vi "Autonomous Independent.vi"   [LabVIEW 2011]
doc: "This VI is called when autonomous begins, and will automatically be terminated when autonomous ends. You can carry out timed or sensor driven robot movement independently without needing to return to the caller."
uses:
  <vilib>/Rock Robotics/WPI/SafetyOutput/WPI_SafetyOutputConfigMenu.ctl
  Robot Global Data.vi
  System Set Points and States.vi
types:
  T1 = typedef "WPI_SafetyOutputConfigMenu.ctl" = enum16{"Enable", "Disable"}
  T2 = typedef "WPI_MotorControlDeviceRef.ctl" = cluster{"DeviceStatus":errorcluster, "Type":enum16{"PWM", "CAN"}, "PWM":cluster{"Digital Module":T3, "PWM Channel":T4, "DeadBand":T5}, "CAN":cluster{"Device Number":u8, "Control Mode":T6, "Semaphore":T7, "Max Vout":dbl}, "Invert":bool, "TransformRef":T8, "InvTransformRef":T8}
  T3 = typedef "FPGA_TypedefDigitalModule.ctl" = enum16{"Digital Module 1", "Digital Module 2"}
  T4 = typedef "FPGA_DIOPWMChannel.ctl" = enum8{"PWM 1", "PWM 2", "PWM 3", "PWM 4", "PWM 5", "PWM 6", "PWM 7", "PWM 8", "PWM 9", "PWM 10", "Invalid"}
  T5 = typedef "WPI_PWMDeadband.ctl" = cluster{"Name":string, "maxPositivePwm":i32, "minPositivePwm":i32, "centerPwm":i32, "maxNegativePwm":i32, "minNegativePwm":i32, "angularRange":u16}
  T6 = typedef "WPI_CANJaguar_ControlMode.ctl" = enum8{"Percent VBus", "Current", "Speed", "Position", "Voltage"}
  T7 = typedef "Semaphore RefNum" = refnum<k1>
  T8 = typedef "WPI_PWMTransform_ConPane.ctl" = refnum<vi>
  T9 = typedef "WPI_DigitalInputDevRef.ctl" = cluster{"DevStatus":errorcluster, "DIO Channel":T10, "Digital Module":T3}
  T10 = typedef "FPGA_DIOChannel.ctl" = enum8{"DIO 1", "DIO 2", "DIO 3", "DIO 4", "DIO 5", "DIO 6", "DIO 7", "DIO 8", "DIO 9", "DIO 10", "DIO 11", "DIO 12", "DIO 13", "DIO 14", "Invalid"}
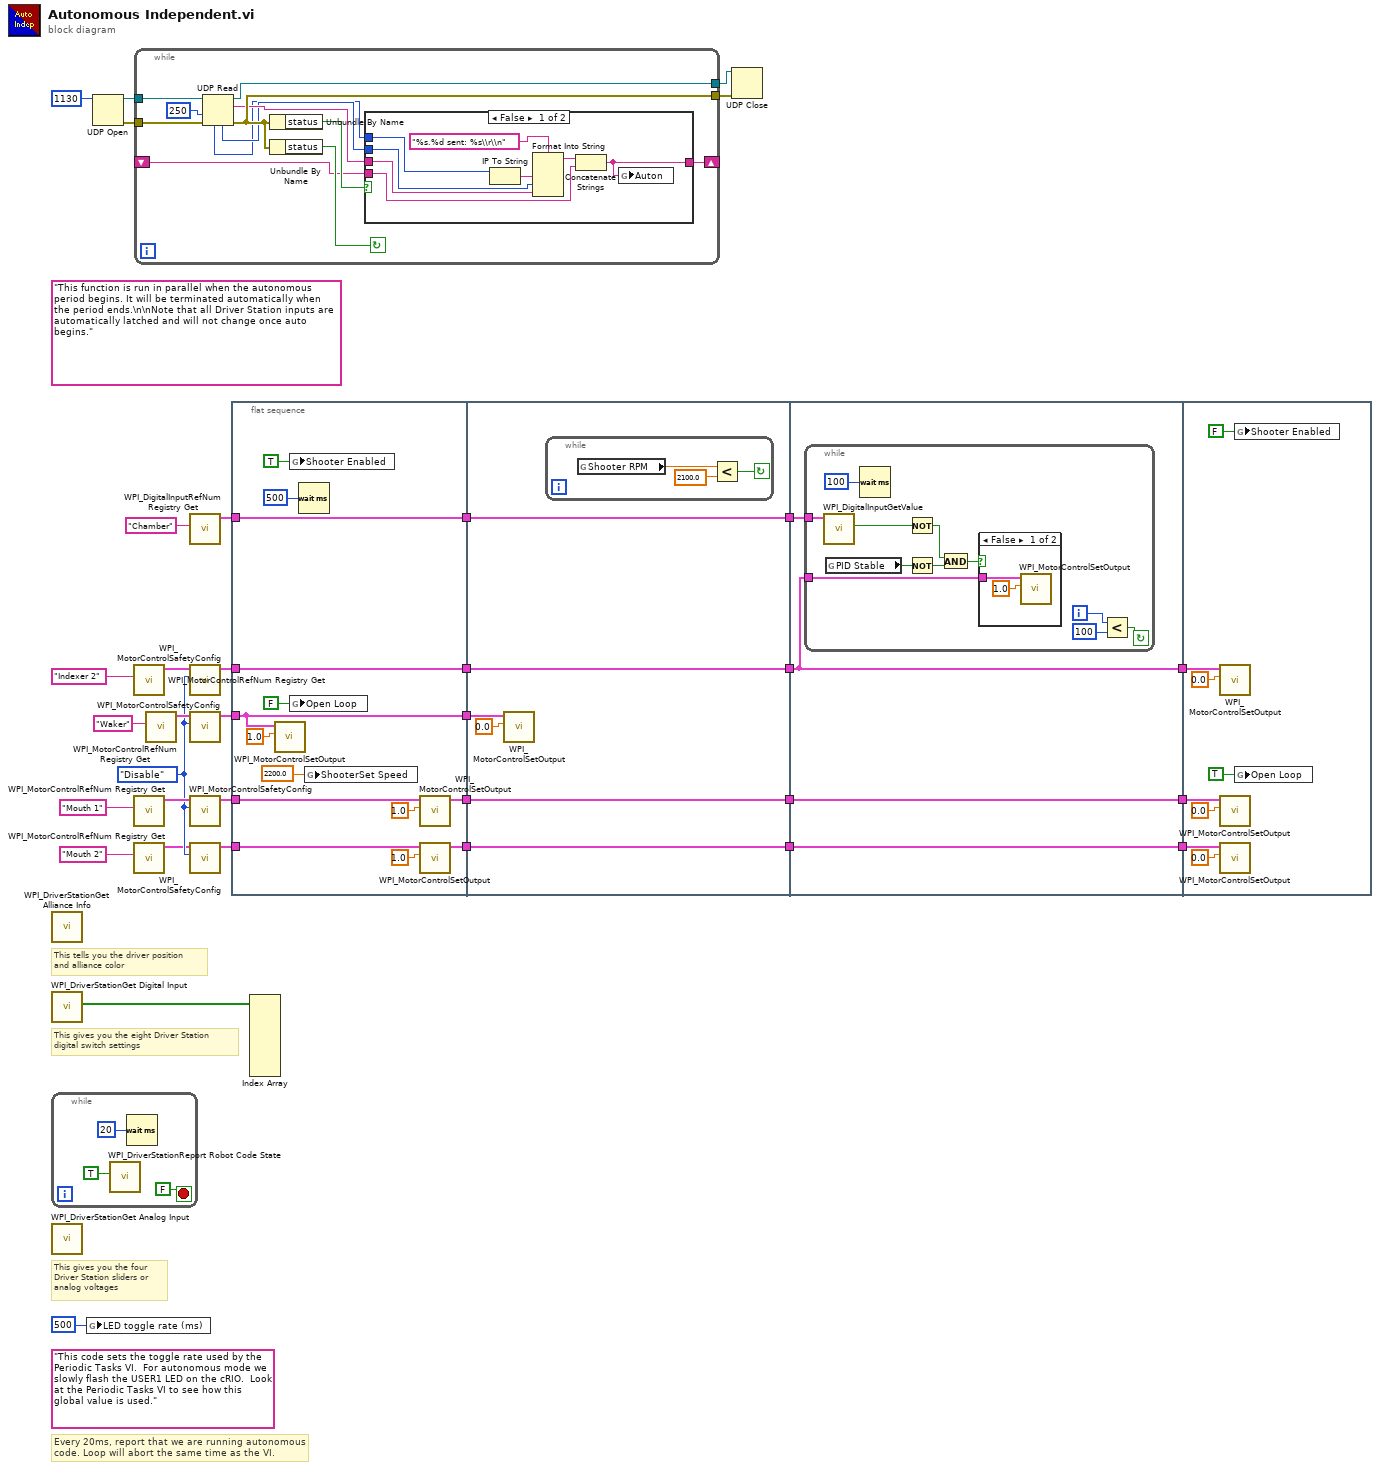
[diagram p0: block diagram]
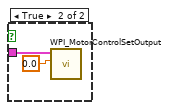
[diagram p2: hidden frame]
diagram:
  w6 = WPI_SafetyOutputConfigMenu."Disable" ("mode")
  (unwired) "This code sets the toggle rate used by the Periodic Tasks VI.  For autonomous mode we slowly flash the USER1 LED on the cRIO.  Look at the Periodic Tasks VI to see how this global value is used."
  (unwired) "This function is run in parallel when the autonomous period begins. It will be terminated automatically when the period ends.\n\nNote that all Driver Station inputs are automatically latched and will not change once auto begins."
  # "Every 20ms, report that we are running autonomous\ncode. Loop will abort the same time as the VI."
  # "This tells you the driver position\nand alliance color"
  # "This gives you the eight Driver Station\ndigital switch settings"
  # "This gives you the four\nDriver Station sliders or\nanalog voltages"
  n1 = call <vilib>:"WPI_DriverStationGet Alliance Info.vi"() -> ()  [unwired: 12 out]
  n2 = call <vilib>:"WPI_DriverStationGet Digital Input.vi"() -> ("Driver Station Digital Input (1-8)"=w20:bool[])  [unwired: 11 out]
  n3 = while {
    stop <- FALSE stop-if-true
    n4 = call <vilib>:"WPI_DriverStationReport Robot Code State.vi"("Autonomous"=TRUE) -> ()  [unwired: 10 in, 1 out]
    n5 = Wait (ms)(milliseconds to wait=u32 20) -> ()  [unwired: 1 out]
  }
  n6 = call <vilib>:"WPI_DriverStationGet Analog Input.vi"() -> ()  [unwired: 12 out]
  n7 = global write "Robot Global Data.vi" "LED toggle rate (ms)"(u32 500 ("LED ms toggle rate")) -> ()
  n8 = UDP Open(11:u16 1130 ("port")) -> (port=w32:refnum<k16>, 0:w34:errorcluster)  [unwired: 4 in, 1 out]
  n9 = call <vilib>:"WPI_MotorControlRefNum Registry Get.vi"("refnum name"="Indexer 2") -> ("MotorControlDevRef"=w16:T2)  [unwired: 9 in, 1 out]
  n10 = call <vilib>:"WPI_MotorControlRefNum Registry Get.vi"("refnum name"="Mouth 1") -> ("MotorControlDevRef"=w11:T2)  [unwired: 9 in, 1 out]
  n11 = call <vilib>:"WPI_MotorControlRefNum Registry Get.vi"("refnum name"="Mouth 2") -> ("MotorControlDevRef"=w5:T2)  [unwired: 9 in, 1 out]
  n12 = while {
    tunnel: w34 -> [w49]
    tunnel: w32 -> [w48]
    tunnel: [w47] -> w31
    tunnel: [w44] -> w30
    shift-right: [w38] -> _
    shift-left: _ -> [w39]
    stop <- w45 continue-if-true
    n13 = UDP Read(connection ID=w48, timeout ms (25000)=250, 8:w49) -> (data out=w42:string, error out=w44:errorcluster, 3:w47:refnum<k16>, 4:w41:u16, 6:w40:u32)  [unwired: 1 in]
    n14 = Unbundle By Name(w44) -> ("status"=w43:bool)
    n15 = Unbundle By Name(w44) -> ("status"=w45:bool)
    n16 = case shown="False" w43 {
      tunnel: w42 -> [w51 _]
      tunnel: w41 -> [w55 _]
      tunnel: w40 -> [w53 _]
      tunnel: w39 -> [w52 w58]
      tunnel: [w50 w58] -> w38
      frame False {
        n17 = IP To String(2:w53) -> (0:w54:string)  [unwired: 1 in]
        n18 = Format Into String(format string="%s.%d sent: %s\\r\\n", w54, w55, w51) -> (resulting string=w57:string)  [unwired: 2 in, 1 out]
        n19 = Concatenate Strings(w57, w52) -> (w50:string)
        n20 = global write "System Set Points and States.vi" "Auton"(w50) -> ()
      }
      frame True {
      }
    }
  }
  n21 = call <vilib>:"WPI_MotorControlRefNum Registry Get.vi"("refnum name"="Waker") -> ("MotorControlDevRef"=w14:T2)  [unwired: 9 in, 1 out]
  n22 = call <vilib>:"WPI_DigitalInputRefNum Registry Get.vi"("refnum name"="Chamber") -> ("DigitalInputDevRef"=w12:T9)  [unwired: 9 in, 1 out]
  n23 = call <vilib>:"WPI_MotorControlSafetyConfig.vi"("mode"=w6, "MotorControlDevRef"=w16) -> ("MotorControlDevRef"=w15:T2)  [unwired: 8 in, 1 out]
  n24 = call <vilib>:"WPI_MotorControlSafetyConfig.vi"("mode"=w6, "MotorControlDevRef"=w14) -> ("MotorControlDevRef"=w13:T2)  [unwired: 8 in, 1 out]
  n25 = call <vilib>:"WPI_MotorControlSafetyConfig.vi"("mode"=w6, "MotorControlDevRef"=w11) -> ("MotorControlDevRef"=w9:T2)  [unwired: 8 in, 1 out]
  n26 = call <vilib>:"WPI_MotorControlSafetyConfig.vi"("mode"=w6, "MotorControlDevRef"=w5) -> ("MotorControlDevRef"=w4:T2)  [unwired: 8 in, 1 out]
  n27 = flat-sequence {
    tunnel: w15 -> [w67]
    tunnel: w13 -> [w65]
    tunnel: w12 -> [w66]
    tunnel: [w67] -> w29
    tunnel: [w66] -> w28
    tunnel: [w65] -> w27
    tunnel: w9 -> [w63]
    tunnel: [w60] -> w26
    tunnel: w4 -> [w62]
    tunnel: [w59] -> w3
    tunnel: w29 -> [w78]
    tunnel: [w78] -> w25
    tunnel: w28 -> [w77]
    tunnel: [w77] -> w24
    tunnel: w27 -> [w76]
    tunnel: [w74] -> w23
    tunnel: w26 -> [w74]
    tunnel: w3 -> [w73]
    tunnel: [w73] -> w2
    tunnel: w25 -> [w84]
    tunnel: w24 -> [w85]
    tunnel: [w84] -> w22
    tunnel: [w83] -> w21
    tunnel: w23 -> [w83]
    tunnel: w2 -> [w82]
    tunnel: [w82] -> w1
    tunnel: w22 -> [w105]
    tunnel: w21 -> [w103]
    tunnel: w1 -> [w101]
    frame #0 {
      n28 = call <vilib>:"WPI_MotorControlSetOutput.vi"("Output"=1.0, "MotorControlDevRef"=w65) -> ()  [unwired: 8 in, 2 out]
      n29 = global write "System Set Points and States.vi" "Shooter Enabled"(TRUE ("Shooter Enabled")) -> ()
      n30 = global write "System Set Points and States.vi" "Open Loop"(FALSE ("Open Loop")) -> ()
      n31 = Wait (ms)(milliseconds to wait=u32 500) -> ()  [unwired: 1 out]
      n32 = global write "System Set Points and States.vi" "ShooterSet Speed"(2200.0) -> ()
      n33 = call <vilib>:"WPI_MotorControlSetOutput.vi"("Output"=1.0, "MotorControlDevRef"=w63) -> ("MotorControlDevRef"=w60:T2)  [unwired: 8 in, 1 out]
      n34 = call <vilib>:"WPI_MotorControlSetOutput.vi"("Output"=1.0, "MotorControlDevRef"=w62) -> ("MotorControlDevRef"=w59:T2)  [unwired: 8 in, 1 out]
    }
    frame #1 {
      n35 = call <vilib>:"WPI_MotorControlSetOutput.vi"("Output"=0.0, "MotorControlDevRef"=w76) -> ()  [unwired: 8 in, 2 out]
      n36 = while {
        stop <- w79 continue-if-true
        n37 = global read "System Set Points and States.vi" "Shooter RPM"() -> (w81:dbl)
        n38 = Less?(x=w81, y=2100.0) -> (x < y?=w79:bool)
      }
    }
    frame #2 {
      n39 = while {
        tunnel: w85 -> [w96]
        tunnel: w84 -> [w95]
        i -> [w93]
        stop <- w91 continue-if-true
        n40 = call <vilib>:"WPI_DigitalInputGetValue.vi"("DigitalInputDevRef"=w96) -> ("Value"=w90:bool)  [unwired: 8 in, 2 out]
        n41 = global read "System Set Points and States.vi" "PID Stable"() -> (w88:bool)
        n42 = Wait (ms)(milliseconds to wait=u32 100) -> ()  [unwired: 1 out]
        n43 = Not(x=w90) -> (.not. x?=w89:bool)
        n44 = Not(x=w88) -> (.not. x?=w87:bool)
        n45 = And(x=w89, y=w87) -> (x .and. y?=w86:bool)
        n46 = case shown="False" w86 {
          tunnel: w95 -> [w98 w100]
          frame False {
            n47 = call <vilib>:"WPI_MotorControlSetOutput.vi"("Output"=1.0, "MotorControlDevRef"=w98) -> ()  [unwired: 8 in, 2 out]
          }
          frame True {
            n48 = call <vilib>:"WPI_MotorControlSetOutput.vi"("Output"=0.0, "MotorControlDevRef"=w100) -> ()  [unwired: 8 in, 2 out]
          }
        }
        n49 = Less?(x=w93, y=100) -> (x < y?=w91:bool)
      }
    }
    frame #3 {
      n50 = call <vilib>:"WPI_MotorControlSetOutput.vi"("Output"=0.0, "MotorControlDevRef"=w105) -> ()  [unwired: 8 in, 2 out]
      n51 = call <vilib>:"WPI_MotorControlSetOutput.vi"("Output"=0.0, "MotorControlDevRef"=w103) -> ()  [unwired: 8 in, 2 out]
      n52 = call <vilib>:"WPI_MotorControlSetOutput.vi"("Output"=0.0, "MotorControlDevRef"=w101) -> ()  [unwired: 8 in, 2 out]
      n53 = global write "System Set Points and States.vi" "Shooter Enabled"(FALSE ("Shooter Enabled")) -> ()
      n54 = global write "System Set Points and States.vi" "Open Loop"(TRUE ("Open Loop")) -> ()
    }
  }
  n55 = Index Array(array=w20) -> ()  [unwired: 8 in, 8 out]
  n56 = UDP Close(connection ID=w31, 8:w30) -> ()  [unwired: 2 out]
